vi "Cleanup.vi"(8 "error in (no error)":errorcluster, 11 "Team Dashboard Panel in":refnum<class "Team Dashboard Panel.lvclass">) -> (0 "error out":errorcluster)   [LabVIEW 2020, in "SB App.lvlib" / "Team Dashboard Panel.lvclass"]
uses:
  Team Dashboard Panel.lvclass
  Team Dashboard Panel.lvclass/Team Dashboard Panel.ctl
  <vilib>/IlluminatedG/IG OOPanel/OOPanel/ArrayPanel/ArrayPanel.lvclass
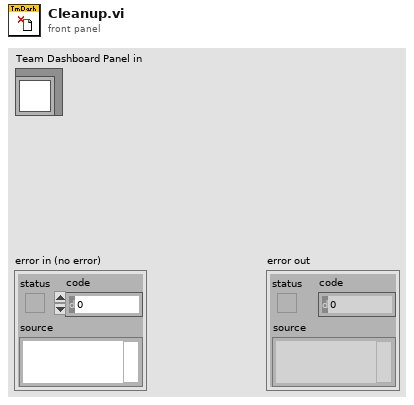
[diagram p1: front panel]
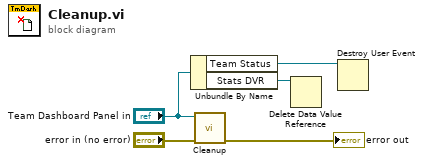
[diagram p0: block diagram]
diagram:
  n1 = Unbundle By Name("Team Dashboard Panel in") -> ("Team Status"=w1:refnum<user-event>, "Stats DVR"=w2:refnum<data-value>)
  n2 = call-parent "Cleanup.vi"("error in (no error)"="error in (no error)", "ArrayPanel in"="Team Dashboard Panel in") -> ("error out"=→"error out":errorcluster)  [unwired: 9 in]
  n3 = Delete Data Value Reference(data value reference=w2) -> ()  [unwired: 1 in, 2 out]
  n4 = Destroy User Event(user event=w1) -> ()  [unwired: 1 in, 1 out]
